vi "4461 Replace AO Ch.vi"(8 "error in (no error)":errorcluster, 10 "Lockin.DAQ (NEW)":refnum<class "Instrument.DAQ.lvclass">, 11 "Lockin.DAQ (OLD)":refnum<class "Instrument.DAQ.lvclass">) -> (0 "error out":errorcluster, 3 "Lockin.DAQ out":refnum<class "Instrument.DAQ.lvclass">)   [LabVIEW 2019, in "Instrument.DAQ.lvclass"]
uses:
  Instrument.DAQ.lvclass
  Instrument.DAQ.lvclass/Instrument.DAQ.ctl
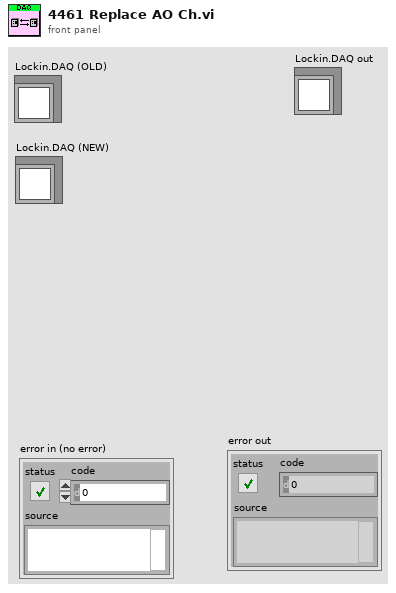
[diagram p1: front panel]
types:
  T1 = typedef "Instrument.DAQ.lvclass/AO-cluster.ctl" = T2[]
  T2 = typedef "Instrument UI.Lockin.lvclass/AO Channel--Cluster.ctl" = cluster{"Enable?":bool, "Channel":i32, "Amplitude":dbl, "Offset":dbl, "Frequency":dbl, "Phase":dbl, "Function":T3, "Sweeping?":bool}
  T3 = typedef "Instrument.DAQ.lvclass/Function-enum.ctl" = enum16{"Sine", "Triangle", "Square"}
  T4 = typedef "Instrument.DAQ.lvclass/REF-cluster.ctl" = T5[]
  T5 = typedef "Instrument UI.Lockin.lvclass/REF Channel--Cluster.ctl" = cluster{"Enable?":bool, "Channel":i32, "Frequency":dbl, "Phase":dbl, "TC":dbl, "Roll-Off":i32}
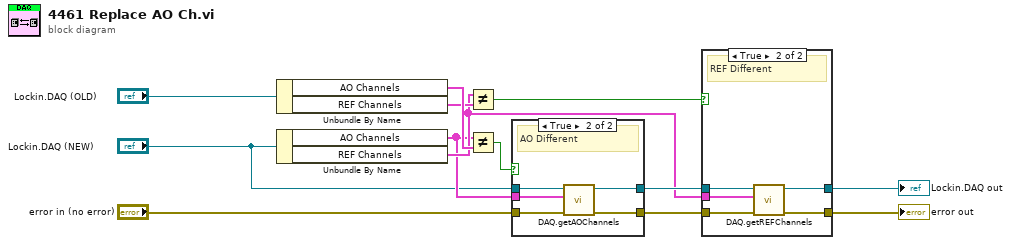
[diagram p0: block diagram]
diagram:
  n1 = Unbundle By Name("Lockin.DAQ (OLD)") -> ("AO Channels"=w12:T1, "REF Channels"=w11:T4)
  n2 = Unbundle By Name("Lockin.DAQ (NEW)") -> ("AO Channels"=w2:T1, "REF Channels"=w3:T4)
  n3 = Not Equal?(x=w3, y=w11) -> (x != y?=w9:bool)
  n4 = Not Equal?(x=w2, y=w12) -> (x != y?=w10:bool)
  n5 = case shown="True" w10 {
    tunnel: [w15 w19] -> w7
    tunnel: "Lockin.DAQ (NEW)" -> [w15 w20]
    tunnel: "error in (no error)" -> [w14 w18]
    tunnel: [w14 w17] -> w5
    tunnel: w2 -> [_ w16]
    frame False {
    }
    frame True {
      # "AO Different"
      n6 = call "DAQ.getAOChannels.vi"("error in (no error)"=w18, "Channels: AO"=w16, "Lockin.DAQ"=w20) -> ("error out"=w17:errorcluster, "Lockin.DAQ"=w19:refnum<class "Instrument.DAQ.lvclass">)  [unwired: 7 in]
    }
  }
  n7 = case shown="True" w9 {
    tunnel: [w22 w26] -> w8
    tunnel: w7 -> [w22 w27]
    tunnel: w5 -> [w21 w25]
    tunnel: [w21 w24] -> w4
    tunnel: w3 -> [_ w23]
    frame False {
    }
    frame True {
      # "REF Different"
      n8 = call "DAQ.getREFChannels.vi"("error in (no error)"=w25, "Channels: REF"=w23, "Lockin.DAQ"=w27) -> ("error out"=w24:errorcluster, "Lockin.DAQ"=w26:refnum<class "Instrument.DAQ.lvclass">)  [unwired: 7 in]
    }
  }
  "Lockin.DAQ out" <- w8
  "error out" <- w4
